vi "randnum_from-20to50.vi"() -> (3 "Numeric":dbl)   [LabVIEW 2017]
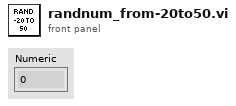
[diagram p1: front panel]
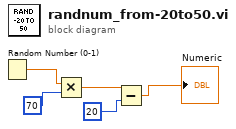
[diagram p0: block diagram]
diagram:
  n1 = Random Number (0-1)() -> (number: 0 to 1=w2:dbl)
  n2 = Multiply(x=w2, y=70) -> (x*y=w3:dbl)
  n3 = Subtract(x=w3, y=20) -> (x-y=→"Numeric":dbl)
